vi "AccessArray.vi"(4 "Sequence Context":T1) -> (0 "error out":errorcluster, 1 "Test Data":T2 {"Numeric Measurement" format="%.2f"})   [LabVIEW 2010]
doc: "This example demonstrates how to use ActiveX to access arrays of data in TestStand from LabVIEW code modules."
uses:
  <vilib>/addons/TestStand/_TSLegacy.llb/LabVIEW Test - Test Data.ctl
  <vilib>/addons/TestStand/_TSLegacy.llb/LabVIEW Test - Sequence Context.ctl
panel:
  out "Array of Data":dbl[](graph)=[0.0, 0.12533323356430426, 0.2486898871648548, 0.3681245526846779, 0.4817536741017153, 0.5877852522924731, 0.6845471059286886, 0.7705132427757893, 0.8443279255020151, 0.9048270524660196, 0.9510565162951535, 0.9822872507286886, 0.9980267284282716, 0.9980267284282716, 0.9822872507286887, 0.9510565162951536, 0.9048270524660195, 0.8443279255020152, 0.7705132427757893, 0.6845471059286888, 0.5877852522924732, 0.4817536741017152, 0.36812455268467814, 0.24868988716485482, 0.12533323356430454, 1.2246063538223773e-16, -0.12533323356430429, -0.24868988716485457, -0.3681245526846779, -0.481753674101715, -0.587785252292473, -0.6845471059286887, -0.7705132427757894, -0.8443279255020149, -0.9048270524660194, -0.9510565162951535, -0.9822872507286887, -0.9980267284282716, -0.9980267284282716, -0.9822872507286887, -0.9510565162951536, -0.9048270524660196, -0.844327925502015, -0.7705132427757896, -0.684547105928689, -0.5877852522924734, -0.4817536741017153, -0.36812455268467786, -0.24868988716485535, -0.12533323356430465, -2.4492127076447545e-16, 0.12533323356430418, 0.24868988716485488, 0.36812455268467736, 0.4817536741017149, 0.5877852522924729, 0.6845471059286886, 0.7705132427757893, 0.8443279255020147, 0.9048270524660194, 0.9510565162951535, 0.9822872507286886, 0.9980267284282716, 0.9980267284282716, 0.9822872507286886, 0.9510565162951536, 0.90482705246602, 0.8443279255020151, 0.7705132427757897, 0.6845471059286884, 0.5877852522924734, 0.4817536741017162, 0.368124552684678, 0.2486898871648555, 0.1253332335643039, 3.673819061467132e-16, -0.12533323356430318, -0.24868988716485477, -0.36812455268467725, -0.48175367410171555, -0.5877852522924728, -0.6845471059286878, -0.7705132427757893, -0.8443279255020146, -0.9048270524660197, -0.9510565162951534, -0.9822872507286885, -0.9980267284282716, -0.9980267284282716, -0.9822872507286886, -0.9510565162951538, -0.90482705246602, -0.8443279255020151, -0.7705132427757897, -0.6845471059286885, -0.5877852522924735, -0.4817536741017163, -0.3681245526846781, -0.2486898871648556, -0.125333233564304]
  in  "stop":bool
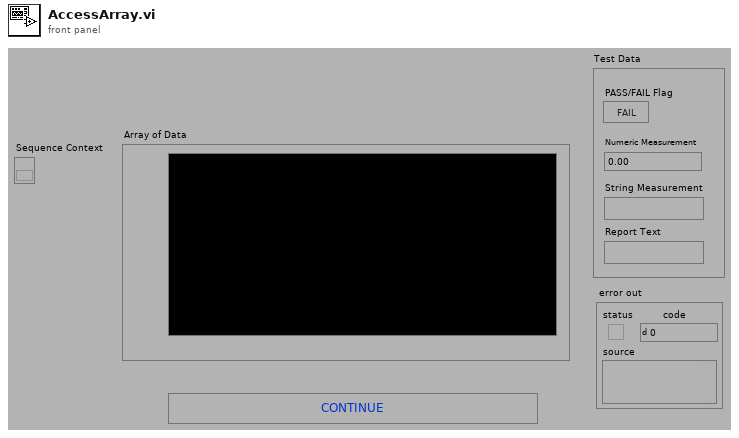
[diagram p1: front panel]
types:
  T1 = typedef "LabVIEW Test - Sequence Context.ctl" = refnum<k7>
  T2 = typedef "LabVIEW Test - Test Data.ctl" = cluster{"PASS/FAIL Flag":bool, "Numeric Measurement":dbl, "String Measurement":string, "Report Text":string}
  T3 = cluster{"Execution":refnum<k7>, "InitTerminationMonitor":refnum<k7>, "Sequence Context Out":refnum<k7>}
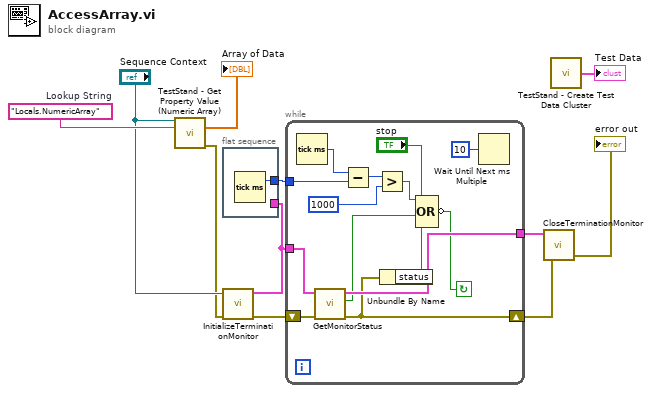
[diagram p0: block diagram]
diagram:
  w10 = "Locals.NumericArray"  # Lookup String
  n1 = call <vilib>:"TestStand - Get Property Value (Numeric Array).vi"("Sequence Context In"="Sequence Context", "Lookup String"=w10) -> ("Value"=→"Array of Data":dbl[], "error out"=w3:errorcluster)  [unwired: 1 in, 11 out]
  n2 = flat-sequence {
    tunnel: [w12] -> w2
    tunnel: w1 -> [_]
    frame #0 {
      n3 = Tick Count (ms)() -> (millisecond timer value=w12:u32)
    }
  }
  n4 = call <vilib>:"InitializeTerminationMonitor.vi"("error in (no error)"=w3, "Sequence Context In"="Sequence Context") -> ("error out"=w6:errorcluster, "StatusMonitor Out"=w1:T3)  [unwired: 8 out]
  n5 = while {
    shift-left: w6 -> [w24]
    shift-right: [w21] -> w5
    tunnel: [w25] -> w7
    tunnel: w1 -> [w26]
    tunnel: w2 -> [w16]
    stop <- w14 continue-if-true
    n6 = Tick Count (ms)() -> (millisecond timer value=w17:u32)
    n7 = call <vilib>:"GetMonitorStatus.vi"("error in"=w24, "StatusMonitor In"=w26) -> ("error out"=w21:errorcluster, "GetTerminationMonitorStatus"=w22:bool, "StatusMonitor Out"=w25:T3)  [unwired: 3 out]
    n8 = Subtract(x=w17, y=w16) -> (x-y=w18:u32)
    n9 = Greater?(x=w18, y=u32 1000) -> (0:w13:bool)
    n10 = Unbundle By Name(w21) -> ("status"=w20:bool)
    n11 = Compound Arithmetic op=OR(w13, "stop", w22, w20) -> (invert w14:bool)
    n12 = Wait Until Next ms Multiple(millisecond multiple=u32 10) -> ()  [unwired: 1 out]
  }
  n13 = call <vilib>:"CloseTerminationMonitor.vi"("error in"=w5, "StatusMonitor In"=w7) -> ("error out"=→"error out":errorcluster)  [unwired: 3 out]
  n14 = call <vilib>:"TestStand - Create Test Data Cluster.vi"() -> ("Test Data"=→"Test Data":T2)  [unwired: 4 in]
